vi "Read Measurement.vi"(4 "Vertical Cross Value (0)":dbl, 6 "Occurrence Value (1)":i32=1, 7 "Slope Type (0: Positive)":i32(ring) items=["Positive", "Negative"], 8 "error in (no error)":errorcluster, 9 "Measurement Type (0: Frequency)":i32(ring) items=["Frequency", "Mean", "Period", "Pulse Duty", "Peak to Peak", "Cycle RMS", "Minimum", "Maximum", "Rise Time", "Fall Time", "Positive Width", "Negative Width", "Amplitude", "Cycle Mean", "High", "Low", "Negative Duty", "Positive Overshoot", "Negative Overshoot", "Cursor Mean", "Burst Width", "Positive Pulse Count", "Negative Pulse Count", "Rising Edge Count", "Falling Edge Count", "Area", "Cycle Area", "RMS", "Cursor RMS"], 10 "Channel (1: Channel 1)":i32(ring)=1 items=["Channel 1"=1, "Channel 2"=2, "Channel 3"=3, "Channel 4"=4], 11 "KS EDU-X 1002G in":refnum<class "KS EDU-X 1002G.lvclass">) -> (0 "error out":errorcluster, 1 "Units":string, 2 "Measurement":dbl, 3 "KS EDU-X 1002G out":refnum<class "KS EDU-X 1002G.lvclass">, 5 "Result Value":dbl)   [LabVIEW 2020, in "Oscilloscope.lvlib" / "KS EDU-X 1002G.lvclass"]
uses:
  KS EDU-X 1002G.lvclass
  C:/Users/ronad/Osciloscopio/Osciloscopio DQMH/Libraries/Oscilloscope/Clases/Osciloscopio/Osciloscopio.lvclass
  Clases/Osciloscopio/Osciloscopio.lvclass/Osciloscopio.ctl
  Clases/Osciloscopio/Read COM.vi
  Clases/Osciloscopio/Write COM.vi
  <instrlib>/Agilent 2000 3000 X-Series/Public/Data/Read Measurement (Current Value).vi
  <instrlib>/Agilent 2000 3000 X-Series/Agilent 2000 3000 X-Series.lvlib
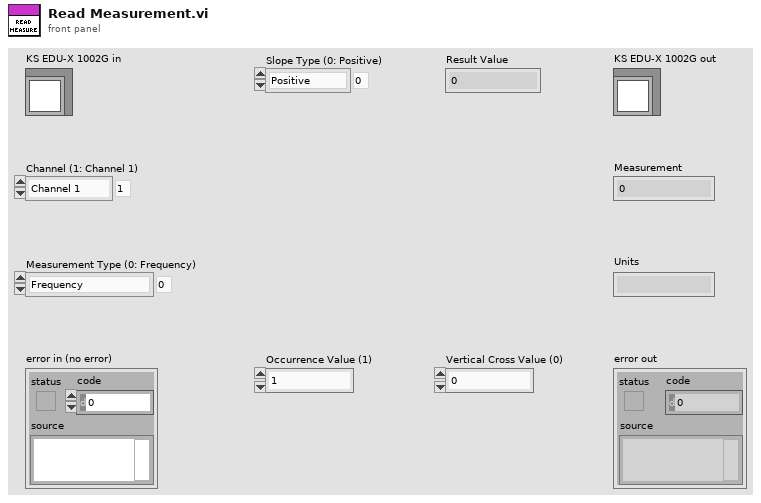
[diagram p1: front panel]
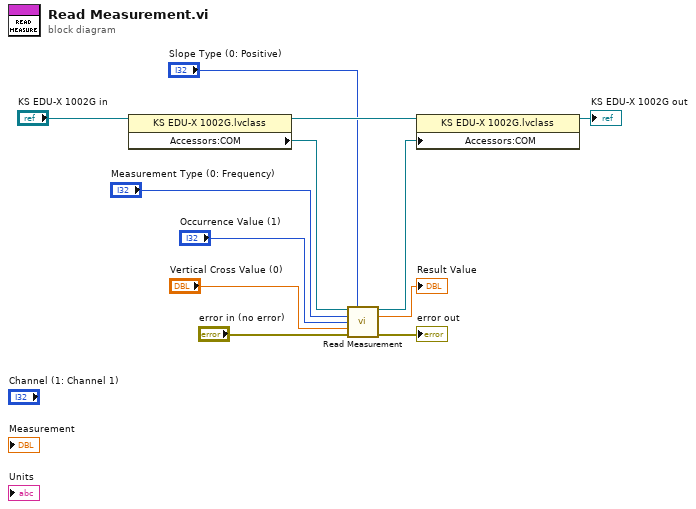
[diagram p0: block diagram]
diagram:
  n1 = property class="KS EDU-X 1002G.lvclass"(reference="KS EDU-X 1002G in") -> (reference out=w10:refnum<class "KS EDU-X 1002G.lvclass">, "Accessors:COM"=w11:refnum<visa-resource-name>)  [unwired: 1 in, 1 out]
  n2 = call-poly <instrlib>:"Read Measurement.vi"("VISA resource name"=w11, "Slope Type (0: Positive)"="Slope Type (0: Positive)", "Measurement Type (0: Peak-Peak)"="Measurement Type (0: Frequency)", "Occurrence Value (1)"="Occurrence Value (1)", "Vertical Cross Value (0)"="Vertical Cross Value (0)", "error in (no error)"="error in (no error)") -> ("VISA resource name out"=w9:refnum<visa-resource-name>, "Result Value"=→"Result Value":dbl, "error out"=→"error out":errorcluster)  [unwired: 7 in]
  n3 = property class="KS EDU-X 1002G.lvclass"(reference=w10, "Accessors:COM"=w9) -> (reference out=→"KS EDU-X 1002G out":refnum<class "KS EDU-X 1002G.lvclass">)  [unwired: 1 in, 1 out]
